vi "getgrat.vi"(2 "error in (no error)":errorcluster) -> (0 "error out":errorcluster, 1 "Grating":i32)   [LabVIEW 2017]
doc: "Queries the grating number in use from the monochromator\n\nReturns No Eror in error out for success, See Error Codes"
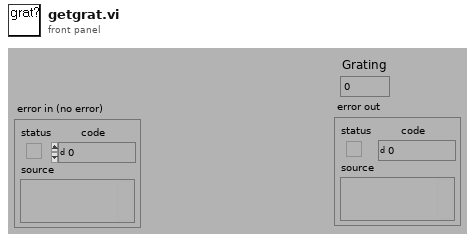
[diagram p1: front panel]
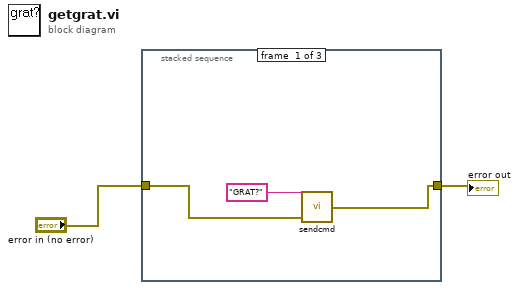
[diagram p0: block diagram]
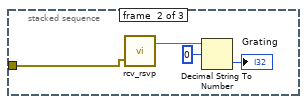
[diagram p2: hidden frame]
diagram:
  n1 = stacked-sequence {
    tunnel: "error in (no error)" -> [w3 w6 _]
    tunnel: [w4 _ _] -> w1
    frame #0 {
      n2 = call "sendcmd.vi"("error in (no error)"=w3, "command in"="GRAT?") -> ("error out"=w4:errorcluster)  [unwired: 1 in]
    }
    frame #1 {
      n3 = call "rcv_rsvp.vi"("error in (no error)"=w6) -> ("response string"=w7:string)  [unwired: 1 in, 1 out]
      n4 = Decimal String To Number(string=w7, offset=0) -> (number=→"Grating":i32)  [unwired: 1 in, 1 out]
    }
    frame #2 {
    }
  }
  "error out" <- w1
